vi "MS SQL_Stn_Count.vi"(6 "Message":refnum<vi>, 8 "error in (no error)":errorcluster, 11 "Ref in":T2={"MS SQL Connection"=refnum, "UDL File"=path "", "Time"="", "DCODE"="", "WIP+1"=0, "MC No?"=0, "POKAYOKE?"=FALSE, "Expected Result"="", "Result [Status]"="", "Clock"=0.0, "RFID"="", "WIP Queue"=refnum, "TS Parameter"={"ProfitCenterCode"="", "LineCode"="", "WorkOrderNumber"="", "Model"="", "Model_with_Prefix"="", "VendorCode"="", "SetParameterDateCode"="", "PokaYoke"=0, "Target"=1, "Live_DateCode"="", "CustomerPartNumber"="", "Hand"="", "sBarcode"=FALSE, "FCA"=0, "Ent_Stamp"=timestamp(0 s since 1904-01-01), "STS_CD"=0.0}, "Data_Queue"=[], "RFID Serial No."=""} {"TS Parameter"."FCA" format="%01d"; "TS Parameter"."Target" min=1 max=100000; "TS Parameter"."PokaYoke" min=0 max=1}) -> (0 "error out":errorcluster, 1 "Pky Status":T1, 3 "Ref Out":T2={"MS SQL Connection"=refnum, "UDL File"=path "", "Time"="", "DCODE"="", "WIP+1"=0, "MC No?"=0, "POKAYOKE?"=FALSE, "Expected Result"="", "Result [Status]"="", "Clock"=0.0, "RFID"="", "WIP Queue"=refnum, "TS Parameter"={"ProfitCenterCode"="", "LineCode"="", "WorkOrderNumber"="", "Model"="", "Model_with_Prefix"="", "VendorCode"="", "SetParameterDateCode"="", "PokaYoke"=0, "Target"=1, "Live_DateCode"="", "CustomerPartNumber"="", "Hand"="", "sBarcode"=FALSE, "FCA"=0, "Ent_Stamp"=timestamp(0 s since 1904-01-01), "STS_CD"=0.0}, "Data_Queue"=[], "RFID Serial No."=""} {"TS Parameter"."FCA" format="%01d"; "TS Parameter"."Target" min=1 max=100000; "TS Parameter"."PokaYoke" min=0 max=1})   [LabVIEW 2020]
uses:
  Controls/TD SQL.ctl
  <vilib>/addons/database/Connection.llb/Conn ObjectReference.ctl
  Controls/WIP_State.ctl
  Controls/TS_Parameter.ctl
  Controls/Poka_Status.ctl
  Controls/PKYK_Status_Enum.ctl
  Controls/Msg_Type.ctl
  MS_Global.vi
  <userlib>/_OpenG.lib/array/array.llb/Search 1D Array (Boolean)__ogtk.vi
  <userlib>/_OpenG.lib/array/array.llb/Index 1D Array Elements (String)__ogtk.vi
  <vilib>/addons/database/NI_Database_API.lvlib
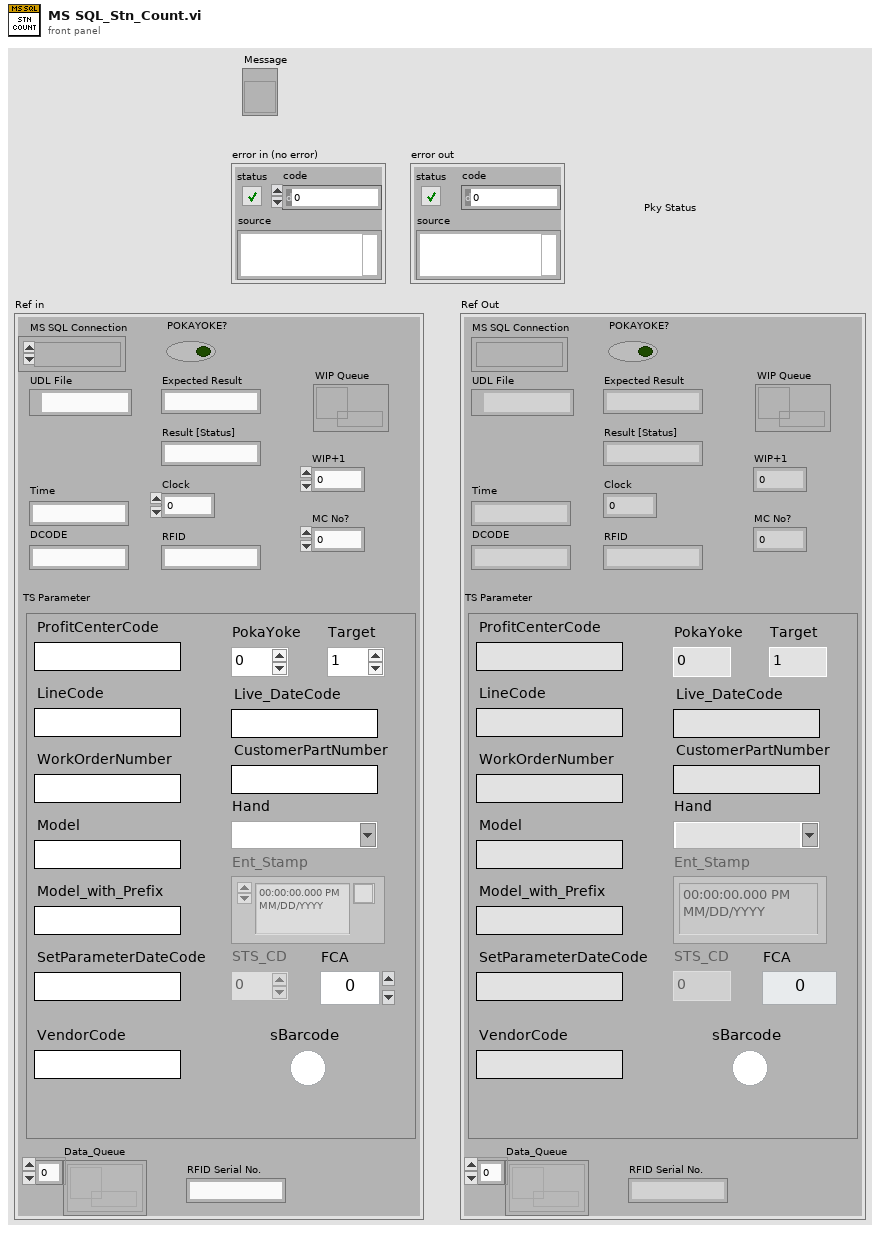
[diagram p1: front panel]
types:
  T1 = typedef "Poka_Status.ctl" = u16
  T2 = typedef "TD SQL.ctl" = cluster{"MS SQL Connection":T3, "UDL File":path, "Time":string, "DCODE":string, "WIP+1":i64, "MC No?":i32, "POKAYOKE?":bool, "Expected Result":string, "Result [Status]":string, "Clock":dbl, "RFID":string, "WIP Queue":refnum<queue>, "TS Parameter":T4, "Data_Queue":refnum<queue>[], "RFID Serial No.":string}
  T3 = typedef "NI_Database_API.lvlib/Conn ObjectReference.ctl" = refnum<k1>
  T4 = typedef "TS_Parameter.ctl" = cluster{"ProfitCenterCode":string, "LineCode":string, "WorkOrderNumber":string, "Model":string, "Model_with_Prefix":string, "VendorCode":string, "SetParameterDateCode":string, "PokaYoke":i32, "Target":i32, "Live_DateCode":string, "CustomerPartNumber":string, "Hand":string, "sBarcode":bool, "FCA":i32, "Ent_Stamp":timestamp, "STS_CD":dbl}
  T5 = typedef "WIP_State.ctl" = enum16{"Open", "Read", "Write", "Read WIP", "Flush", "Close"}
  T6 = typedef "Msg_Type.ctl" = enum16{"Normal", "Pass", "Fail", "Fault", "User", "Bypass", "Fail Save"}
  T7 = typedef "PKYK_Status_Enum.ctl" = enum16{"PKYK_Wait", "PKYK_Done"}
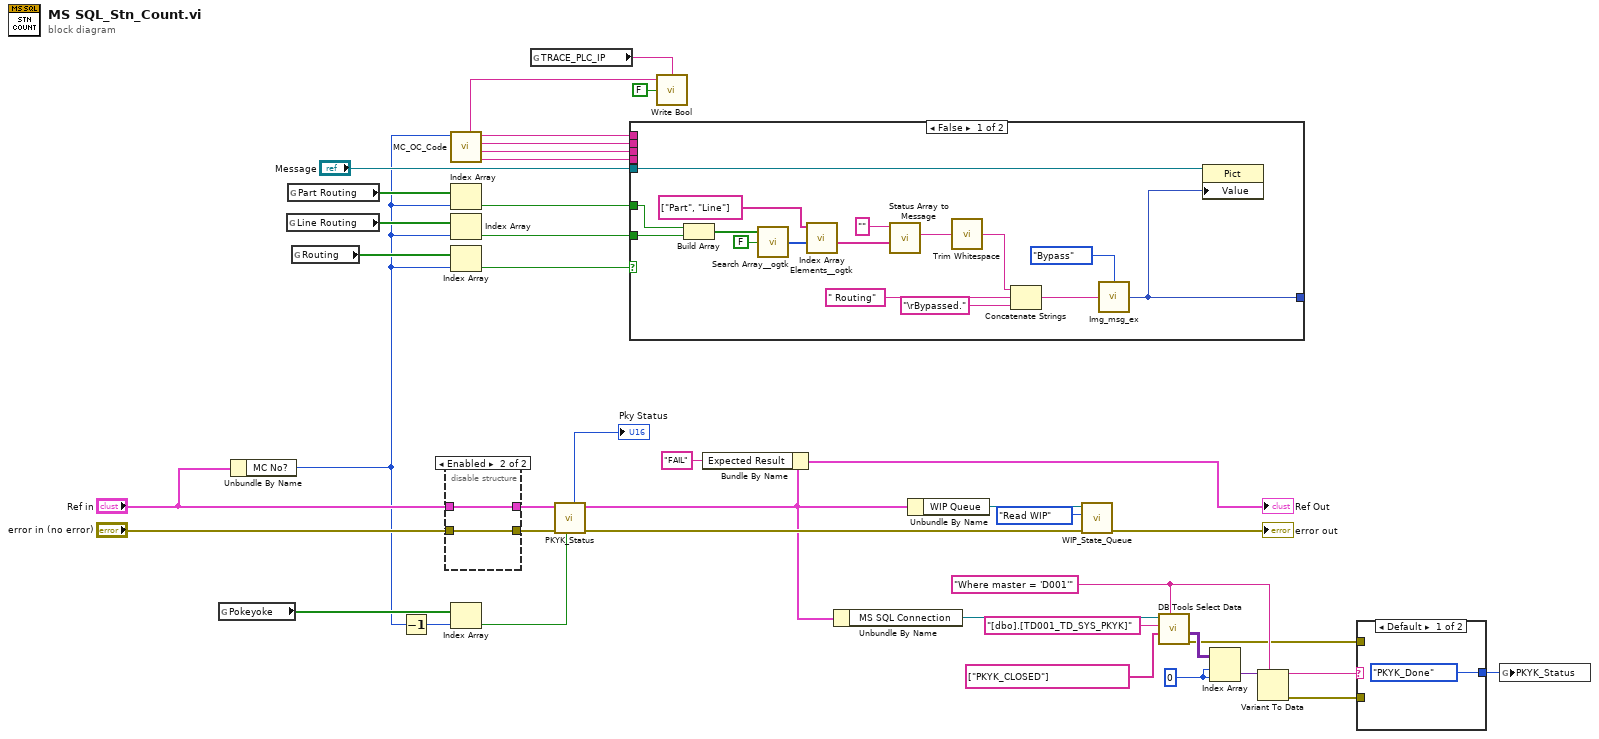
[diagram p0: block diagram]
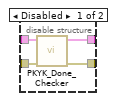
[diagram p2: hidden frame]
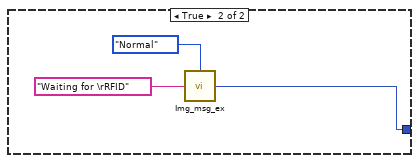
[diagram p3: hidden frame]
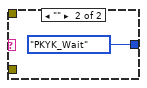
[diagram p4: hidden frame]
diagram:
  w35 = 0 ("index (row)")
  w33 = "Where master = 'D001'" ("condition")
  n1 = global read "MS_Global.vi" "Pokeyoke"() -> (w9:bool[])
  n2 = Unbundle By Name("Ref in") -> ("MC No?"=w3:i32)
  n3 = global read "MS_Global.vi" "Line Routing"() -> (w19:bool[])
  n4 = global read "MS_Global.vi" "Part Routing"() -> (w20:bool[])
  n5 = global read "MS_Global.vi" "Routing"() -> (w23:bool[])
  n6 = Decrement(x=w3) -> (x-1=w8:i32)
  n7 = disable-structure shown="Enabled" {
    disable-tunnel: "error in (no error)" -> [w45 w46]
    disable-tunnel: [w44 w47] -> w40
    disable-tunnel: [w43 w46] -> w39
    disable-tunnel: "Ref in" -> [w42 w47]
    frame Disabled {
      n8 = call "PKYK_Done_Checker.vi"("error in (no error)"=w45, "Ref in"=w42) -> ("error out"=w43:errorcluster, "Ref out"=w44:T2)  [unwired: 5 in, 3 out]
    }
    frame Enabled {
    }
  }
  n9 = call "MC_OC_Code.vi"("index"=w3) -> ("Code Query"=w6:string, "TS CODE TAG"=w5:string, "Machine Code"=w21:string, "Operation Code"=w4:string, "Data Saved Tag"=w12:string)  [unwired: 4 in, 2 out]
  n10 = Index Array(array=w20, index=w3) -> (element=w17:bool)
  n11 = Index Array(array=w19, index=w3) -> (element=w18:bool)
  n12 = Index Array(array=w23, index=w3) -> (element=w22:bool)
  n13 = Index Array(array=w9, index=w8) -> (element=w7:bool)
  n14 = global read "MS_Global.vi" "TRACE_PLC_IP"() -> (w13:string)
  n15 = call "PKYK_Status.vi"("PokaYoke?"=w7, "error in (no error)"=w39, "Ref in"=w40) -> ("error out"=w27:errorcluster, "Ref out"=w2:T2, "Pky Status"=→"Pky Status":T1)  [unwired: 5 in, 1 out]
  n16 = case shown="False" w22 {
    tunnel: w21 -> [_ _]
    tunnel: w18 -> [w62 _]
    tunnel: w17 -> [w63 _]
    tunnel: [w48 w64] -> _
    tunnel: "Message" -> [w49 _]
    tunnel: w6 -> [_ _]
    tunnel: w5 -> [_ _]
    tunnel: w4 -> [_ _]
    frame False {
      n17 = Build Array(w63, w62) -> (w61:bool[])
      n18 = call-poly <userlib>:"Search Array__ogtk.vi"("Array"=w61, "Element Data"=FALSE) -> ("Indices of Elements"=w59:i32[])  [unwired: 7 in]
      n19 = call-poly <userlib>:"Index Array Elements__ogtk.vi"("indices"=w59, "array"=string[] ["Part", "Line"] ("Status Array")) -> ("elements"=w57:string[])  [unwired: 9 in]
      n20 = call <userlib>:"Status Array to Message.vi"("Status Array"=w57, "Message"="") -> ("Message"=w55:string)  [unwired: 9 in]
      n21 = call <vilib>:"Trim Whitespace.vi"("string"=w55) -> ("trimmed string"=w52:string)  [unwired: 1 in]
      n22 = Concatenate Strings(w52, " Routing" ("string"), "\rBypassed." ("string")) -> (w50:string)
      n23 = call "Img_msg_ex.vi"("Msg Type"=Msg_Type."Bypass", "Message In"=w50) -> ("Message"=w48:picture)  [unwired: 2 in]
      n24 = property class="Pict"(reference=w49, "Value"=w48) -> ()  [unwired: 1 in, 2 out]
    }
    frame True {
      n25 = call "Img_msg_ex.vi"("Msg Type"=Msg_Type."Normal", "Message In"="Waiting for \rRFID") -> ("Message"=w64:picture)  [unwired: 2 in]
    }
  }
  n26 = call "Write Bool.vi"("Network Path"=w13, "Int"=FALSE, "Tag Name"=w12) -> ()  [unwired: 2 in]
  n27 = Bundle By Name(cluster=w2, "Expected Result"="FAIL") -> (→"Ref Out":T2)
  n28 = Unbundle By Name(w2) -> ("MS SQL Connection"=w28:T3)
  n29 = Unbundle By Name(w2) -> ("WIP Queue"=w1:refnum<queue>)
  n30 = call "WIP_State_Queue.vi"("error in (no error)"=w27, "State In"=WIP_State."Read WIP", "Queue In"=w1) -> ("error out"=→"error out":errorcluster)  [unwired: 6 in, 2 out]
  n31 = call <vilib>:"DB Tools Select Data.vi"("condition"=w33, "columns"=string[] ["PKYK_CLOSED"], "table"="[dbo].[TD001_TD_SYS_PKYK]", "connection reference"=w28) -> ("error out"=w24:errorcluster, "data"=w36:variant[][])  [unwired: 2 in, 1 out]
  n32 = Index Array(array=w36, index (row)=w35, index (col)=w35) -> (element=w34:variant)
  n33 = Variant To Data(type=w33, Variant=w34) -> (data=w30:string, error out=w31:errorcluster)  [unwired: 1 in]
  n34 = case shown="Default" w30 {
    tunnel: w31 -> [_ _]
    tunnel: [PKYK_Status_Enum."PKYK_Done" ("PKYK_Status") PKYK_Status_Enum."PKYK_Wait" ("PKYK_Status")] -> w29
    tunnel: w24 -> [_ _]
    frame Default {
    }
    frame "" {
    }
  }
  n35 = global write "MS_Global.vi" "PKYK_Status"(w29) -> ()
